vi "SelfTest.vi"(0 "comport":string, 11 "error in (no error)":errorcluster, 12 "Clear Errors":bool=TRUE, 13 "Open Ser(t)":bool, 14 "Close Ser(t)":bool) -> (3 "Pass?(t)":bool, 4 "output":string, 15 "error out":errorcluster)   [LabVIEW 2018]
uses:
  <vilib>/regexp/Match Regular Expression.xnode
panel:
  out "after match":string
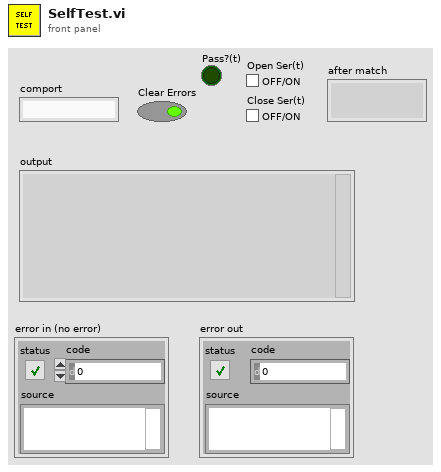
[diagram p1: front panel]
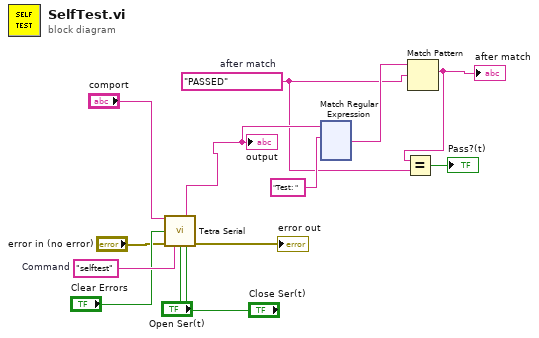
[diagram p0: block diagram]
diagram:
  w2 = "PASSED"  # after match
  w13 = "selftest"  # Command
  n1 = call "Tetra Serial.vi"("COMPORT"="comport", "ClearErrorIn(t)"="Clear Errors", "error in (no error)"="error in (no error)", "Command"=w13, "Open Ser(t)"="Open Ser(t)", "Close Ser(t)"="Close Ser(t)") -> ("output"=w6:string, "error out"=→"error out":errorcluster)  [unwired: 6 in, 2 out]
  "output" <- w6
  n2 = xnode "Match Regular Expression"("input string"=w6, "regular expression"="Test: ") -> ("after match"=w3:string)  [unwired: 4 in, 4 out]
  n3 = Match Pattern(string=w3, regular expression=w2) -> (match substring=w1:string)  [unwired: 1 in, 3 out]
  "after match" <- w1
  n4 = Equal?(x=w1, y=w2) -> (x = y?=→"Pass?(t)":bool)
